vi "JogPositive.vi"(0 "CmdLib In":refnum<k24>, 5 "DeviceKey In":string, 7 "Device Address In":i32, 9 "Motor":i32, 11 "error in (no error)":errorcluster) -> (4 "CmdLib Out":refnum<k24>, 6 "DeviceKey Out":string, 8 "Device Address Out":i32, 15 "error out":errorcluster)   [LabVIEW 2009]
uses:
  C:/Code/Apps/Utilities/Picomotor/PicomotorApp/Install/Samples/LabVIEW/Model 8743/LabVIEW 2009/CmdLib.dll
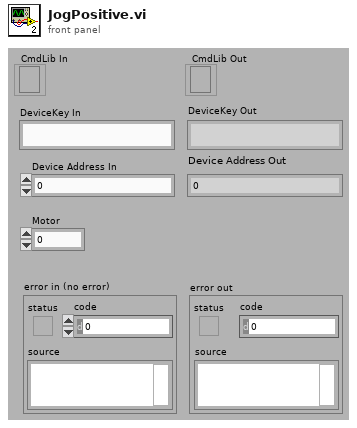
[diagram p1: front panel]
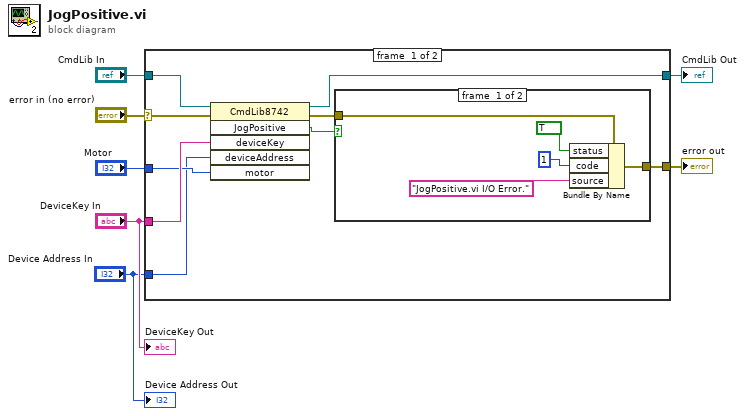
[diagram p0: block diagram]
diagram:
  n1 = case shown="No Error" "error in (no error)" {
    selector: "error in (no error)" -> [w13 w23]
    tunnel: "CmdLib In" -> [w16 w24]
    tunnel: [w15 w24] -> w6
    tunnel: "Motor" -> [w9 _]
    tunnel: "DeviceKey In" -> [w14 _]
    tunnel: [w10 w23] -> w3
    tunnel: "Device Address In" -> [w8 _]
    frame #0 {
      n2 = invoke class="CmdLib8742" method="JogPositive"(reference=w16, error in=w13, "deviceKey"=w14, "deviceAddress"=w8, "motor"=w9) -> (reference out=w15:refnum<k24>, error out=w11:errorcluster, "JogPositive"=w12:bool)  [unwired: 1 in, 3 out]
      n3 = case shown="False" w12 {
        tunnel: w11 -> [w21 w22]
        tunnel: [w20 w22] -> w10
        frame #0 {
          n4 = Bundle By Name(cluster=w21, "status"=TRUE, "code"=1, "source"="JogPositive.vi I/O Error.") -> (w20:errorcluster)
        }
        frame #1 {
        }
      }
    }
    frame #1 {
    }
  }
  "error out" <- w3
  "CmdLib Out" <- w6
  "DeviceKey Out" <- "DeviceKey In"
  "Device Address Out" <- "Device Address In"
